vi "Write On Board Memory (NVM).vi"(0 "Session Handle in":T1, 5 "Address":u16=171 format="%x", 7 "Bytes to Write":u8[](array[numeric]), 11 "error in (no error)":errorcluster) -> (4 "Session Handle out":T1, 15 "error out":errorcluster)   [LabVIEW 2015, in "PAS.lvclass"]
uses:
  PAS.lvclass
  Typedefs/Session Handle.ctl
panel:
  out "Whole Payload":u8[](array[numeric])
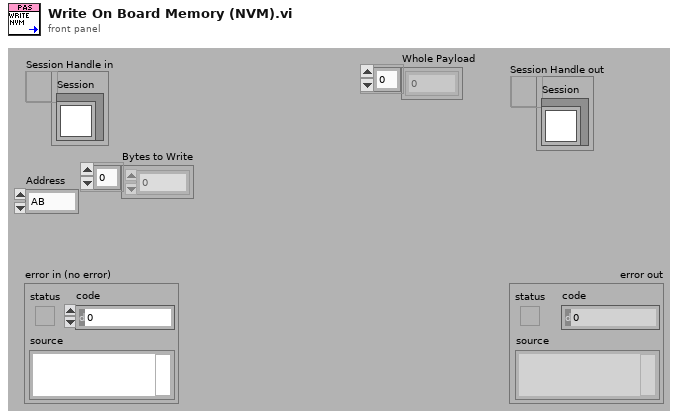
[diagram p1: front panel]
types:
  T1 = typedef "PAS.lvclass/Session Handle.ctl" = refnum<data-value>
  T2 = typedef "XNET Frame CAN.ctl" = cluster{"timestamp":timestamp, "payload":u8[], "identifier":u32, "type":T3, "extended?":bool, "echo?":bool}
  T3 = typedef "XNET Frame Type CAN.ctl" = u8
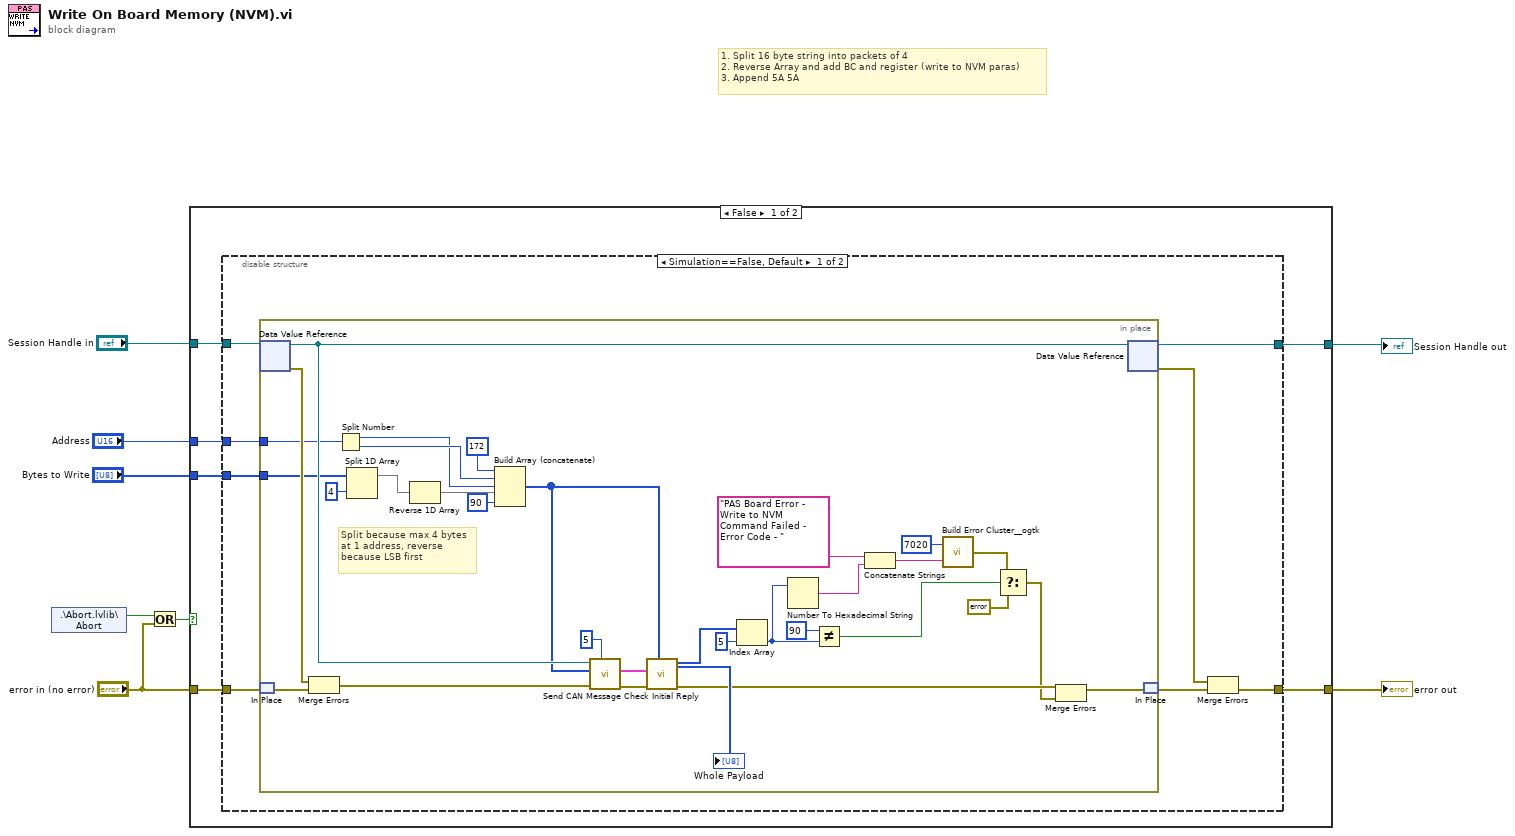
[diagram p0: block diagram]
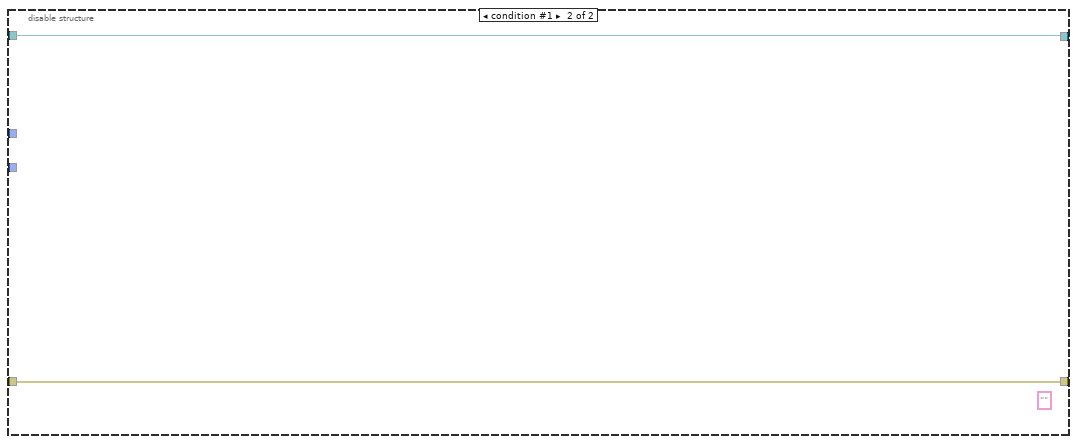
[diagram p2: hidden frame]
diagram:
  # "1. Split 16 byte string into packets of 4\n2. Reverse Array and add BC and register (write to NVM paras)\n3. Append 5A 5A"
  n1 = shared-variable ".\\Abort.lvlib\\Abort"() -> (w5:bool)  [unwired: 1 in, 1 out]
  n2 = Or(x=w5, y="error in (no error)") -> (x .or. y?=w3:bool)
  n3 = case shown="False" w3 {
    tunnel: [w14 w58] -> w7
    tunnel: [w13 w57] -> w6
    tunnel: "Session Handle in" -> [w12 w58]
    tunnel: "error in (no error)" -> [w11 w57]
    tunnel: "Address" -> [w10 _]
    tunnel: "Bytes to Write" -> [w9 _]
    frame False {
      n4 = disable-structure shown="Simulation==False, Default" {
        disable-tunnel: [w22 w56] -> w14
        disable-tunnel: [w19 w55] -> w13
        disable-tunnel: w12 -> [w18 w56]
        disable-tunnel: w11 -> [w17 w55]
        disable-tunnel: w10 -> [w16 _]
        disable-tunnel: w9 -> [w15 _]
        frame condition #0 (active) {
          n5 = in-place {
            in-place-border: w16 -> [w42]
            in-place-border: w15 -> [w30]
            # "Split because max 4 bytes\nat 1 address, reverse \nbecause LSB first"
            n6 = in-place-dvr #1(w18) -> (w51:refnum<class "PAS.lvclass">, w54:errorcluster)
            n7 = in-place-match #2(w17) -> (w53:errorcluster)
            n8 = Merge Errors(w54, w53) -> (w52:errorcluster)
            n9 = Split Number(x=w42) -> (hi(x)=w40:u8, lo(x)=w41:u8)
            n10 = Split 1D Array(array=w30, index=4) -> (first subarray=w28:u8[])  [unwired: 1 out]
            n11 = Reverse 1D Array(array=w28) -> (reversed array=w27:u8[])
            n12 = Build Array (concatenate)(u8 172, w41, w40, w27, u8 90) -> (w46:u8[])
            n13 = call "Send CAN Message.vi"("Number of Retries"=5, "error in (no error)"=w52, "payload"=w46, "Pas In"=w51) -> ("error out"=w25:errorcluster, "Reply"=w47:T2[])  [unwired: 5 in, 1 out]
            n14 = call "Check Initial Reply.vi"("Write Message"=w46, "error in (no error)"=w25, "Reply"=w47) -> ("error out"=w24:errorcluster, "Data Packet"=w39:u8[], "Whole Payload"=→"Whole Payload":u8[])  [unwired: 5 in, 1 out]
            n15 = Index Array(array=w39, index=5) -> (element=w35:u8)
            n16 = Number To Hexadecimal String(2:w35) -> (0:w34:string)  [unwired: 1 in]
            n17 = Not Equal?(x=u8 90, y=w35) -> (x != y?=w32:bool)
            n18 = Concatenate Strings("PAS Board Error - Write to NVM Command Failed - Error Code - " ("string"), w34) -> (w33:string)
            n19 = call <userlib>:"Build Error Cluster__ogtk.vi"("String to Prepend to source (\"\")"=w33, "code"=7020) -> ("error out"=w44:errorcluster)
            n20 = Select(t=w44, s=w32, f=errorcluster {"status"=FALSE, "code"=0, "source"=""}) -> (s? t:f=w23:errorcluster)
            n21 = Merge Errors(w24, w23) -> (w50:errorcluster)
            n22 = in-place-dvr #1(w51) -> (w22:T1, w20:errorcluster)
            n23 = in-place-match #2(w50) -> (w21:errorcluster)
          }
          n24 = Merge Errors(w20, w21) -> (w19:errorcluster)
        }
        frame condition #1 {
          (unwired) "" ("string")
        }
      }
    }
    frame True {
    }
  }
  "Session Handle out" <- w7
  "error out" <- w6
